vi "MARS_Scan_Data_Analysis_global.vi"() -> ()   [LabVIEW 2015]
panel:
  out "Calculated FoM":dbl[](array[numeric])
  out "Channel Index":dbl
  out "Fit Histogram":i32[][][](array[numeric])
  out "Ratio Graph":i32[][][](array[numeric])
  out "FoM Y max":i32
  out "FoM X max":i32
  out "2nd Period":dbl[](array[numeric])
  out "1st Period":dbl[](array[numeric])
  out "FoM Graph":dbl[][](array[numeric])
  out "Scan Total Int":i32[][](array[numeric])
  out "Scan Tail Int":i32[][](array[numeric])
  in  "Channels":string[][](array[string])
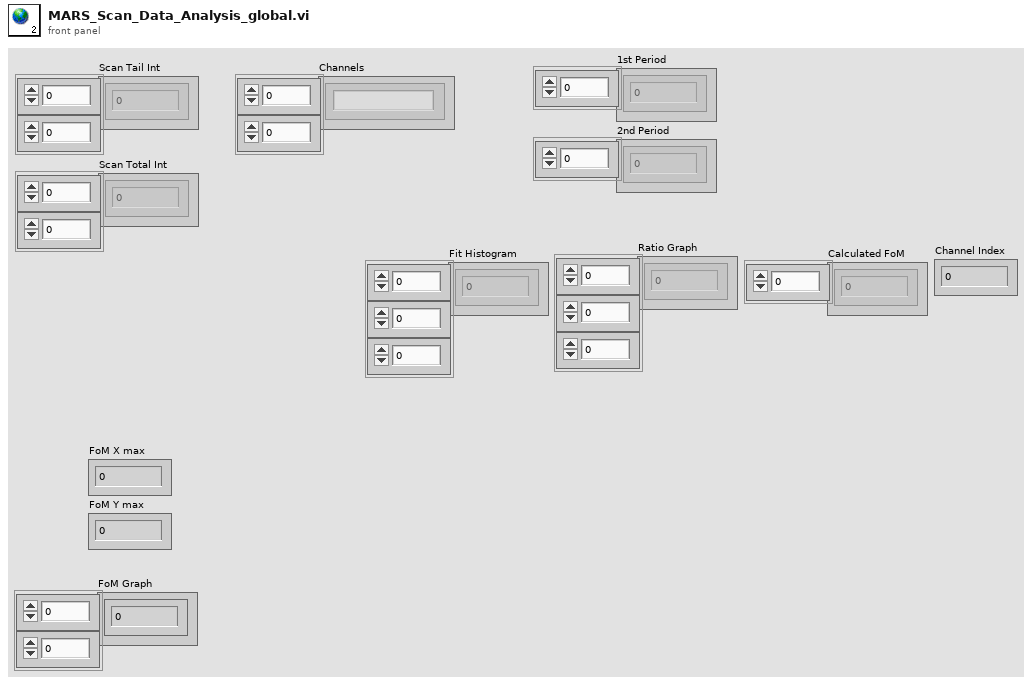
[diagram p1: front panel]
diagram:
